vi "A1 With All Zeros.vi"(11 "DUT Serial #":i32) -> (3 "output array":u8[](array[numeric]))   [LabVIEW 2013]
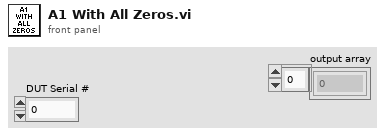
[diagram p1: front panel]
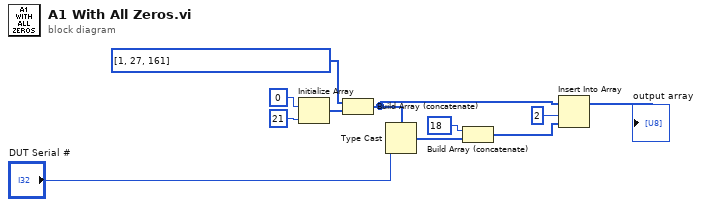
[diagram p0: block diagram]
diagram:
  n1 = Initialize Array(u8 0, 21 ("dimension size")) -> (w5:u8[])
  n2 = Build Array (concatenate)(u8[] [1, 27, 161] ("initialized array"), w5) -> (w6:u8[])
  n3 = Type Cast(type=w6, x="DUT Serial #") -> (*(type *) &x=w4:u8[])
  n4 = Build Array (concatenate)(u8 18, w4) -> (w8:u8[])
  n5 = Insert Into Array(array=w6, index=2, new element=w8) -> (→"output array":u8[])
